vi "Position Minimise Button.vi"(8 "Error In":errorcluster, 11 "Minimise Button Refnum":refnum<vi>) -> (0 "Error Out":errorcluster)   [LabVIEW 2014]
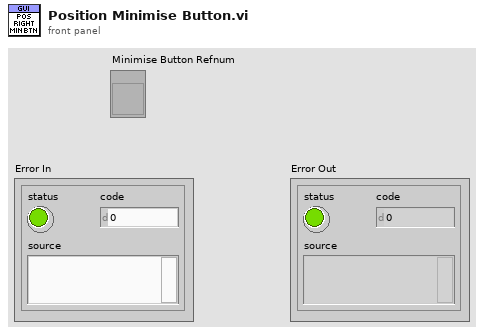
[diagram p1: front panel]
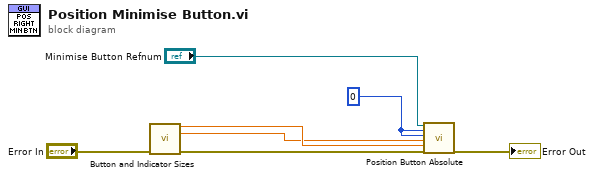
[diagram p0: block diagram]
diagram:
  w4 = 0 ("Left Offset (px)")
  n1 = call "Button and Indicator Sizes.vi"("error in (no error)"="Error In") -> ("Button Width"=w6:dbl, "Button Height"=w5:dbl, "error out"=w7:errorcluster)  [unwired: 10 in, 2 out]
  n2 = call "Position Button Absolute.vi"("Button Ref"="Minimise Button Refnum", "Left Offset (px)"=w4, "Top Offste (px)"=w4, "Height (px)"=w5, "Width (px)"=w6, "Error In"=w7) -> ("Error Out"=→"Error Out":errorcluster)  [unwired: 13 in]
